vi "take the notice.vi"(5 "数组":string[][](array[string])) -> (3 "Original array":string[](array[string]), 4 "Target":dbl, 6 "Min":dbl, 8 "Pace Rate":string, 10 "Max":dbl, 13 "notice":string, 14 "pace amp":string, 15 "Pluse Width":dbl)   [LabVIEW 2016]
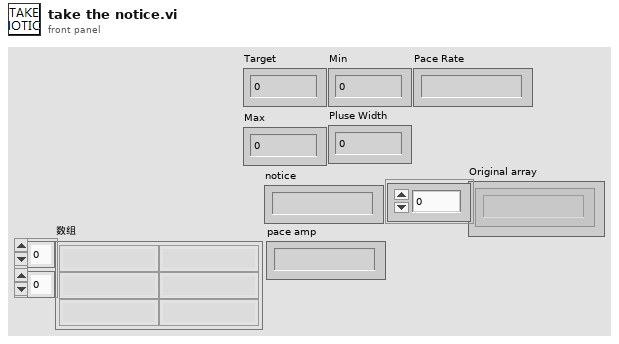
[diagram p1: front panel]
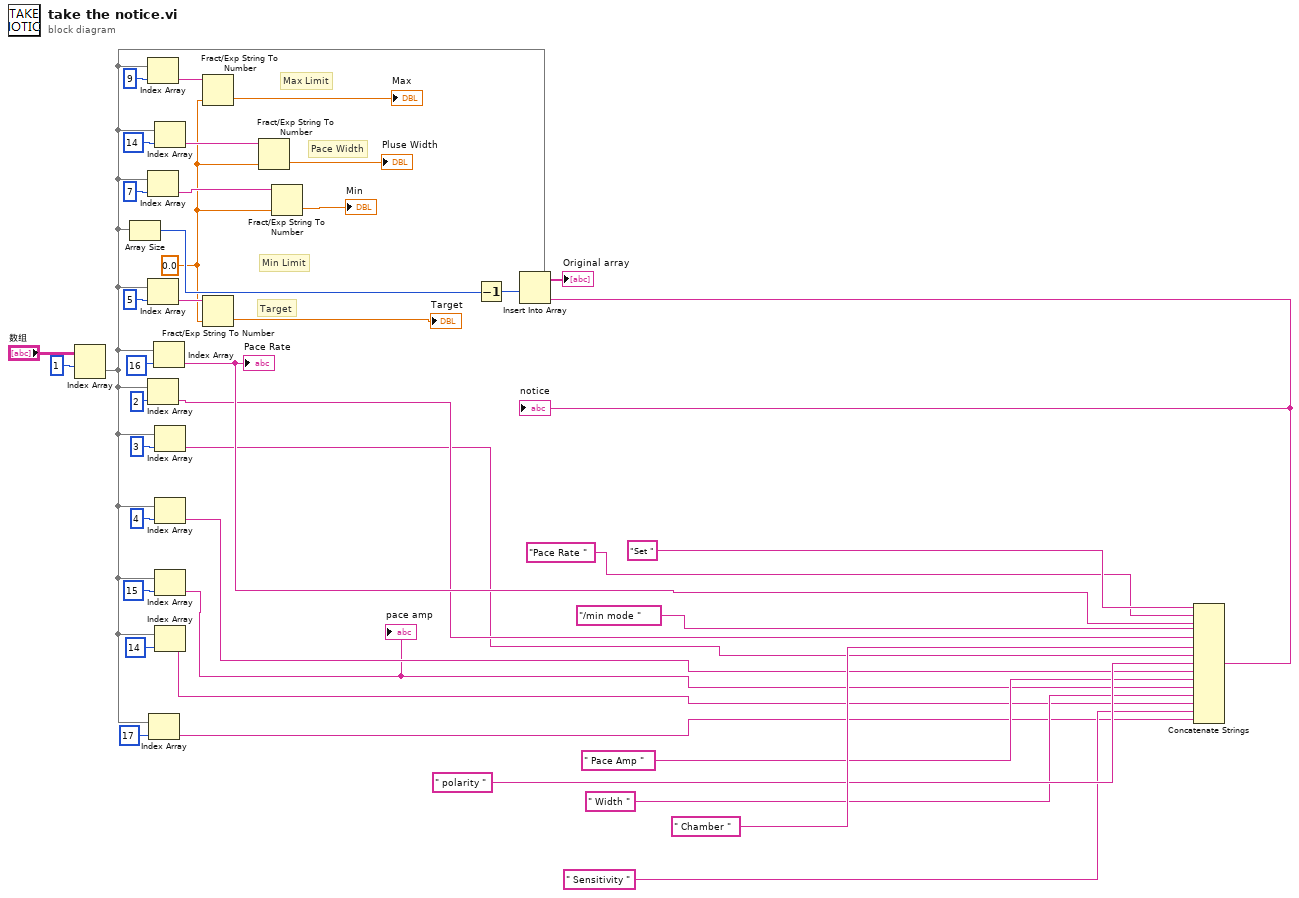
[diagram p0: block diagram]
diagram:
  w21 = 0.0 ("默认(0 I32)")
  # "Pace Width"
  # "Target"
  # "Min Limit"
  # "Max Limit"
  n1 = Index Array(array="数组", index (row)=1 ("索引 (行)")) -> (element=w4:string[])  [unwired: 1 in]
  n2 = Array Size(array=w4) -> (size(s)=w25:i32)
  n3 = Index Array(array=w4, index=9 ("索引")) -> (element=w38:string)
  n4 = Index Array(array=w4, index=7 ("索引")) -> (element=w39:string)
  n5 = Index Array(array=w4, index=5 ("索引")) -> (element=w36:string)
  n6 = Index Array(array=w4, index=2 ("索引")) -> (element=w14:string)
  n7 = Index Array(array=w4, index=17 ("索引")) -> (element=w1:string)
  n8 = Index Array(array=w4, index=16 ("索引")) -> (element=w16:string)
  "Pace Rate" <- w16
  n9 = Index Array(array=w4, index=14 ("偏移量")) -> (element=w34:string)
  n10 = Index Array(array=w4, index=3 ("索引")) -> (element=w12:string)
  n11 = Index Array(array=w4, index=4 ("索引")) -> (element=w10:string)
  n12 = Index Array(array=w4, index=15 ("索引")) -> (element=w8:string)
  "pace amp" <- w8
  n13 = Index Array(array=w4, index=14 ("索引")) -> (element=w5:string)
  n14 = Fract/Exp String To Number(string=w38, default (0 dbl)=w21) -> (number=→"Max":dbl)  [unwired: 2 in, 1 out]
  n15 = Fract/Exp String To Number(string=w36, default (0 dbl)=w21) -> (number=→"Target":dbl)  [unwired: 2 in, 1 out]
  n16 = Fract/Exp String To Number(string=w34, default (0 dbl)=w21) -> (number=→"Pluse Width":dbl)  [unwired: 2 in, 1 out]
  n17 = Fract/Exp String To Number(string=w39, default (0 dbl)=w21) -> (number=→"Min":dbl)  [unwired: 2 in, 1 out]
  n18 = Decrement(x=w25) -> (x-1=w24:i32)
  n19 = Concatenate Strings("Set " ("字符串"), "Pace Rate " ("字符串"), w16, "/min mode " ("字符串"), w14, " Chamber " ("字符串"), w12, " polarity " ("字符串"), w10, " Pace Amp " ("字符串"), w8, " Width " ("字符串"), w5, " Sensitivity " ("字符串"), w1) -> (w23:string)
  "notice" <- w23
  n20 = Insert Into Array(array=w4, index=w24, new element=w23) -> (→"Original array":string[])
